vi "SwapEDVRsForTypedefs.vi"() -> ()   [LabVIEW 2020]
uses:
  <vilib>/Utility/traverseref.llb/TRef TravTarget.ctl
  <vilib>/numeric/LVNumericRepresentation.ctl
  image/ARGB Image.ctl
  image/Greyscale Image.ctl
  <vilib>/Utility/traverseref.llb/VI Scripting - Traverse.lvlib
  <vilib>/Utility/Data Type/NI_Data Type.lvlib
  image/image.lvlib
panel:
  out "Of":i32
  out "Current":i32
  out "Path":path
  out "Array":errorcluster[](array[cluster])
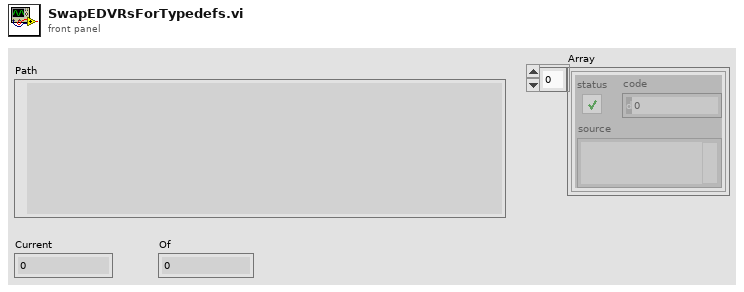
[diagram p1: front panel]
types:
  T1 = enum32{"Invalid", "Standard", "Closed", "Hidden", "Minimized", "Maximized"}
  T2 = typedef "TRef TravTarget.ctl" = enum16{"FP", "BD", "Other"}
  T3 = enum32{"not a typedef", "typedef", "strict typedef", "class private data"}
  T4 = typedef "LVNumericRepresentation.ctl" = enum32{"Extended Precision", "Double Precision", "Single Precision", "Long", "Word", "Byte", "Unsigned Long", "Unsigned Word", "Unsigned Byte", "Complex Extended", "Complex Double", "Complex Single", "Quad", "Unsigned Quad", "Fixed-Point"}
  T5 = typedef "NI_Data Type.lvlib/Memory Info.ctl" = cluster{"Type":T6, "Size":u32}
  T6 = typedef "NI_Data Type.lvlib/Memory Type.ctl" = enum16{"Variable", "Fixed", "Bounded"}
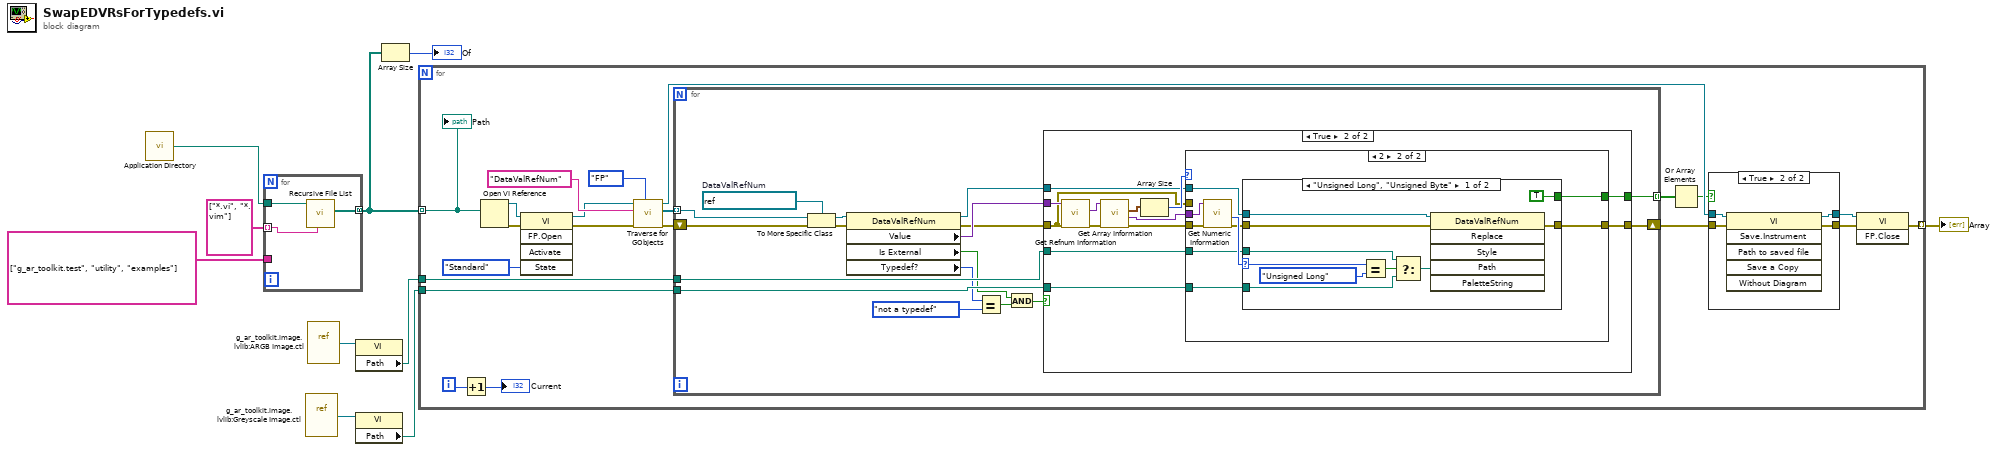
[diagram p0: block diagram]
diagram:
  n1 = call <vilib>:"Application Directory.vi"() -> ("Application Directory"=w10:path)
  n2 = for {
    tunnel: string[] ["g_ar_toolkit.test", "utility", "examples"] ("Folders to Exclude") -> [_]
    tunnel: string[] ["*.vi", "*.vim"] ("Folders to Exclude") -> [w12] mode=indexing
    tunnel: w10 -> [w13]
    tunnel: [w11] -> w2 mode=concatenating
    n3 = call <vilib>:"Recursive File List.vi"("pattern"=w12, "Folder Path"=w13) -> ("All Files in Dir"=w11:path[])  [unwired: 5 in, 4 out]
  }
  n4 = vi-ref "g_ar_toolkit.image.lvlib:Greyscale Image.ctl"() -> (w8:refnum<vi>)
  n5 = vi-ref "g_ar_toolkit.image.lvlib:ARGB Image.ctl"() -> (w9:refnum<vi>)
  n6 = property class="VI"(reference=w9) -> ("Path"=w7:path)  [unwired: 1 in, 2 out]
  n7 = property class="VI"(reference=w8) -> ("Path"=w6:path)  [unwired: 1 in, 2 out]
  n8 = Array Size(array=w2) -> (size(s)=→"Of":i32)
  n9 = for {
    tunnel: w2 -> [w34] mode=indexing
    tunnel: w7 -> [w28]
    tunnel: w6 -> [w27]
    tunnel: [w18] -> w5 mode=indexing
    i -> [w15]
    n10 = Increment(x=w15) -> (x+1=→"Current":i32)
    n11 = Open VI Reference(vi path=w34) -> (vi reference=w33:refnum<vi>, error out=w17:errorcluster)  [unwired: 5 in]
    n12 = invoke class="VI" method="FP.Open"(reference=w33, error in=w17, "State"=T1."Standard") -> (reference out=w26:refnum<vi>, error out=w16:errorcluster)  [unwired: 2 in, 3 out]
    n13 = call <vilib>:"Traverse for GObjects.vi"("Traverse Target"=TRef_TravTarget."FP", "error in (no error)"=w16, "Class Name"="DataValRefNum", "VI Refnum"=w26) -> ("error out"=w29:errorcluster, "References"=w30:refnum<vi>[], "dup VI Refnum"=w24:refnum<vi>)  [unwired: 4 in, 1 out]
    n14 = for {
      tunnel: w30 -> [w57] mode=indexing
      tunnel: w28 -> [w50]
      tunnel: w27 -> [w49]
      shift-right: [w47] -> w21
      shift-left: w29 -> [w53]
      tunnel: [w41] -> w23 mode=indexing
      w56 = refnum<vi> refnum  # DataValRefNum
      n15 = To More Specific Class(target class=w56, reference=w57, error in=w53) -> (specific class reference=w55:refnum<vi>, error out=w52:errorcluster)
      n16 = property class="DataValRefNum"(reference=w55, error in=w52) -> (reference out=w51:refnum<vi>, error out=w48:errorcluster, "Value"=w54:variant, "Is External"=w43:bool, "Typedef?"=w46:T3)
      n17 = Equal?(x=w46, y=T3."not a typedef") -> (x = y?=w42:bool)
      n18 = And(x=w43, y=w42) -> (x .and. y?=w44:bool)
      n19 = case shown="True" w44 {
        tunnel: w54 -> [_ w71]
        tunnel: w51 -> [_ w64]
        tunnel: w50 -> [_ w63]
        tunnel: w49 -> [_ w62]
        tunnel: w48 -> [w58 w60]
        tunnel: [w58 w61] -> w47
        tunnel: [_ w59] -> w41
        frame False {
        }
        frame True {
          n20 = call <vilib>:"Get Refnum Information.vi"("error in (no error)"=w60, "variant"=w71) -> ("error out"=w68:errorcluster, "strict type"=w70:variant)  [unwired: 6 in, 2 out]
          n21 = call <vilib>:"Get Array Information.vi"("error in (no error)"=w68, "variant"=w70) -> ("error out"=w67:errorcluster, "array element data type"=w69:variant, "array lengths"=w66:T5[])  [unwired: 6 in, 1 out]
          n22 = Array Size(array=w66) -> (size(s)=w65:i32)
          n23 = case shown="2" w65 {
            tunnel: w69 -> [_ w81]
            tunnel: w67 -> [_ w80]
            tunnel: w64 -> [_ w77]
            tunnel: w63 -> [_ w76]
            tunnel: w62 -> [_ w75]
            tunnel: [w72 w74] -> w61
            tunnel: w60 -> [w72 _]
            tunnel: [_ w73] -> w59
            frame Default {
            }
            frame 2 {
              n24 = call <vilib>:"Get Numeric Information.vi"("error in (no error)"=w80, "variant"=w81) -> ("error out"=w78:errorcluster, "representation"=w79:T4)  [unwired: 6 in, 2 out]
              n25 = case shown="\"Unsigned Long\", \"Unsigned Byte\"" w79 {
                selector: w79 -> [w89 _]
                tunnel: w78 -> [w90 w92]
                tunnel: w77 -> [w91 _]
                tunnel: w76 -> [w86 _]
                tunnel: w75 -> [w85 _]
                tunnel: [w83 w92] -> w74
                tunnel: [TRUE _] -> w73
                frame "Unsigned Long", "Unsigned Byte" {
                  n26 = Equal?(x=w89, y=LVNumericRepresentation."Unsigned Long") -> (x = y?=w87:bool)
                  n27 = Select(t=w86, s=w87, f=w85) -> (s? t:f=w84:path)
                  n28 = invoke class="DataValRefNum" method="Replace"(reference=w91, error in=w90, "Path"=w84) -> (error out=w83:errorcluster)  [unwired: 3 in, 5 out]
                }
                frame Default {
                }
              }
            }
          }
        }
      }
    }
    n29 = Or Array Elements(Boolean array=w23) -> (logical OR=w22:bool)
    n30 = case shown="True" w22 {
      tunnel: w24 -> [w35 w40]
      tunnel: w21 -> [w36 w39]
      tunnel: [w35 w38] -> w20
      tunnel: [w36 w37] -> w19
      frame False {
      }
      frame True {
        n31 = invoke class="VI" method="Save.Instrument"(reference=w40, error in=w39) -> (reference out=w38:refnum<vi>, error out=w37:errorcluster)  [unwired: 4 in, 4 out]
      }
    }
    n32 = invoke class="VI" method="FP.Close"(reference=w20, error in=w19) -> (error out=w18:errorcluster)  [unwired: 1 in, 2 out]
    "Path" <- w34
  }
  "Array" <- w5
